vi "Window Comparison.vi"() -> ()   [LabVIEW 2010]
doc: "This VI is used to demonstrate the effect of different window functions upon the spectral leakage and low power freqency components of a signal."
uses:
  <vilib>/Analysis/4window.llb/windowTd.ctl
  <vilib>/measure/maspectr.llb/FFT Power Spectrum for N Chan.vi
  <vilib>/measure/NI_MAPro.lvlib
  <vilib>/Analysis/NI_AALPro.lvlib
panel:
  out "Power Spectrum":cluster{"f0":dbl, "df":dbl, "magnitude":dbl[]}[](graph)=[{"f0"=0.0, "df"=1.0, "magnitude"=[-124.1751058373542, -121.13513758298744, -121.04674254070572, -120.90139130147163, -120.70184950660021, -120.4516362912143, -120.15474721632286, -119.81538139357082, -119.43770325848809, -119.02565646304703, -118.58283491900558, -118.11240678765495, -117.61708195919539, -117.0991117628995, -116.56031017833426, -116.00208758694967, -115.42549025871809, -114.83124082124473, -114.21977665062707, -113.59128440951838, -112.94572985272337, -112.28288260850888, -111.60233599546437, -110.90352211751781, -110.18572255543572, -109.44807497004957, -108.68957588923833, -107.90907987456065, -107.10529517249748, -106.27677584755415, -105.42191027644408, -104.53890574697934, -103.62576875027956, -102.68028036961206, -101.69996594374675, -100.68205789832162, -99.62345027411698, -98.5206430009276, -97.36967332386469, -96.16603091496, -94.90455199278048, -93.5792860707239, -92.1833265180739, -90.7085925655272, -89.14554510684852, -87.48281062482066, -85.70667508309265, -83.80038965903157, -81.74319727265596, -79.50893265081362, -77.06394868660806, -74.36393534729245, -71.34882905910446, -67.93423079359103, -63.99595070698343, -59.33964451276823, -53.63348773495808, -46.22884860135584, -35.49862598039451, -12.538597719535238, -3.3068667017160718, -6.4718206580262425, -28.099138539831067, -41.89347763201883, -50.503546856045254, -56.877338492895234, -61.963331522426735, -66.2069680824894, -69.87995537585789, -69.42951944375393, -62.313348426517905, -68.64789111316674, -80.51401763572983, -82.80836943344987, -84.81279857131192, -86.65729225400504, -88.37465396711826, -89.98359184719408, -91.49777512871867, -92.92807128495059, -94.2834408641184, -95.57142153203343, -96.79843898860452, -97.97002633237325, -99.09098728441205, -100.165521673258, -101.1973240562493, -102.18966249313182, -103.14544227261875, -104.06725801235694, -104.95743664052716, -105.81807313810978, -106.6510604744758, -107.4581148423591, -108.24079705696988, -109.00053080261591, -109.73861826993095, -110.45625362163356, -111.15453463886374, -111.83447283746116, -112.49700228807168, -113.14298733692583, -113.77322938535407, -114.38847286548837, -114.9894105215889, -115.5766880932836, -116.15090847961386, -116.71263545156476, -117.26239697121866, -117.80068816515816, -118.32797399671021, -118.84469167010687, -119.35125280119163, -119.84804537868074, -120.33543554231103, -120.81376919508655, -121.28337347152097, -121.74455807294514, -122.19761648788884, -122.64282710653832, -123.08045424111178, -123.51074906186751, -123.93395045607555, -124.35028581883688, -124.75997177970198, -125.1632148746169, -125.56021216445208, -125.95115180889975, -126.33621359494916, -126.71556942981516, -127.08938379504264, -127.45781417102245, -127.82101142978769, -128.1791202007523, -128.53227921375282, -128.88062161485857, -129.22427526570416, -129.56336301902527, -129.89800298045301, -130.22830874930548, -130.55438964584712, -130.87635093206134, -131.19429399733144, -131.50831656127366, -131.81851284256575, -132.12497372712798, -132.42778692495105, -132.7270371169389, -133.0228060950118, -133.31517289129974, -133.60421390401575, -133.89000301319814, -134.17261169109617, -134.4521091078739, -134.72856222806476, -135.0020359079417, -135.27259298004606, -135.54029434084245, -135.8051990277102, -136.0673642984266, -136.32684569329058, -136.58369712500158, -136.83797091414112, -137.08971787479618, -137.3389873620221, -137.5858273315044, -137.83028439067246, -138.07240385123893, -138.31222977771716, -138.54980503079713, -138.78517131635516, -139.01836922222444, -139.24943826165918, -139.478416911193, -139.7053426466115, -139.93025197873203, -140.15318048594614, -140.37416284818175, -140.59323287623275, -140.81042354077957, -141.02576700189334, -141.2392946361118, -141.4510370617037, -141.6610241613996, -141.86928511277793, -142.07584840369356, -142.28074185791914, -142.483992655868, -142.68562735853408, -142.88567191681955, -143.08415170231268, -143.28109151728637, -143.47651561575393, -143.67044771848697, -143.8629110295719, -144.0539282524225, -144.24352160475738, -144.431712831396, -144.61852321890476, -144.80397361171842, -144.98808441974336, -145.1708756360107, -145.35236684339583, -145.5325772323706, -145.71152560552503, -145.8892303949039, -146.06570966571508, -146.24098113376738, -146.41506216755542, -146.58796980481273, -146.75972075422638, -146.93033141296564, -147.09981786390102, -147.26819590045824, -147.43548101168403, -147.60168841453992, -147.76683304143387, -147.93092956156843, -148.09399237373233, -148.25603563199058, -148.41707323198509, -148.57711883559443, -148.73618585914346, -148.89428749748961, -149.0514367127429, -149.20764625749496, -149.36292866143202, -149.51729625611, -149.6707611575352, -149.82333529904795, -149.9750304115177, -150.125858034163, -150.27582953481837, -150.4249560927558, -150.5732487138425, -150.72071823604801, -150.86737532923135, -151.01323049989048, -151.15829409882457, -151.3025763228256, -151.44608720967113, -151.5888366545089, -151.73083441170797, -151.87209009575957, -152.01261317634646, -152.15241299481323, -152.29149875949037, -152.42987955427094, -152.56756433208255, -152.70456192925553, -152.84088106013726, -152.97653032731174, -153.11151820843295, -153.2458530897144, -153.37954322543285, -153.51259678729724, -153.645021827412, -153.77682629940782, -153.90801807014378, -154.03860489156355, -154.16859442078814, -154.297994277555, -154.42681190437577, -154.55505471423885, -154.68273002263447, -154.80984505159046, -154.93640696126272, -155.06242280680107, -155.1878995912301, -155.31284421983273, -155.43726354300745, -155.5611643189456, -155.68455325535066, -155.80743697809953, -155.92982204851444, -156.05171496612618, -156.17312216066736, -156.2940500070311, -156.4145048149012, -156.5344928315363, -156.65402025195718, -156.7730932174993, -156.89171780289058, -157.00990004204607, -157.12764591254404, -157.24496133777103, -157.36185219883018, -157.47832432363407, -157.59438349337324, -157.71003544570368, -157.82528587844814, -157.94014043807178, -158.05460473752296, -158.16868434411612, -158.2823847835679, -158.39571155703294, -158.50867010817984, -158.621265871078, -158.7335042170598, -158.84539050873965, -158.9569300533994, -159.06812815720016, -159.17899006349944, -159.28952100577783, -159.39972618773655, -159.50961078616334, -159.61917994074602, -159.72843878791122, -159.8373924134828, -159.94604591619043, -160.05440432451513, -160.1624726837545, -160.27025601040685, -160.37775930121828, -160.48498753744693, -160.5919456715788, -160.69863865011925, -160.80507140935055, -160.91124884929033, -161.0171758896533, -161.12285740177512, -161.22829828651413, -161.33350338274414, -161.43847757092217, -161.5432256889789, -161.6477525772953, -161.75206307548777, -161.85616199720897, -161.96005417870816, -162.06374442975874, -162.16723755636502, -162.270538396736, -162.37365172534734, -162.47658236739863, -162.57933512730958, -162.6819148077118, -162.78432621977902, -162.88657416961715, -162.9886634783187, -163.09059900120357, -163.19238539686467, -163.2940277286696, -163.395530647562, -163.49689907261245, -163.59813782096313, -163.69925176615436, -163.80024574808377, -163.901124661947, -164.00189337926753, -164.10255679265657, -164.20311979575402, -164.3035873219207, -164.40396429955373, -164.50425568046768, -164.60446638650893, -164.70460143352153, -164.80466578456029, -164.90466445297545, -165.0046024543232, -165.10448481853496, -165.20431665651734, -165.30410293685438, -165.4038488348927, -165.5035594377934, -165.60323986632395, -165.70289527979156, -165.8025308490354, -165.902151751014, -166.00176321081292, -166.10137045679858, -166.20097871960036, -166.30059330525074, -166.4002194740553, -166.4998625659141, -166.59952790049562, -166.69922084209676, -166.79894674812257, -166.8987110446178, -166.99851913465955, -167.09837642826753, -167.1982884040054, -167.29826053310828, -167.3982982866537, -167.49840718821974, -167.59859272778644, -167.69886047166955, -167.79921594423993, -167.89966469275805, -168.00021229453077, -168.10086434194093, -168.20162636701187, -168.30250394388145, -168.4035027068691, -168.5046281860337, -168.60588597566147, -168.70728161197218, -168.80882068148227, -168.91050867688188, -169.0123511118843, -169.1143535166961, -169.21652128779388, -169.31885988465908, -169.42137466391597, -169.52407093732975, -169.6269540104788, -169.7300290787213, -169.8333012583385, -169.936775605551, -170.04045714285007, -170.14435066809898, -170.24846097914164, -170.35279265258796, -170.4573502952991, -170.5621381219311, -170.66716044353166, -170.77242117456504, -170.8779241627027, -170.98367302507282, -171.0896710874559, -171.19592147231293, -171.30242698937437, -171.40919024382862, -171.51621339879216, -171.62349822909803, -171.7310463832929, -171.83885868730476, -171.94693595044146, -172.0552782093128, -172.1638850589407, -172.27275556913153, -172.38188815021238, -172.4912806012415, -172.6009299794752, -172.7108326963813, -172.8209841038539, -172.93137898052328, -173.04201112773544, -173.15287288382228, -173.26395642711663, -173.37525174021863, -173.48674741812613, -173.59843449204186, -173.71029531974932, -173.82231761578305, -173.93448394918724, -174.0467762268345, -174.15917448253055, -174.2716563870087, -174.3841980792969, -174.49677339554017, -174.60935352674574, -174.72190764756215, -174.83440208790205, -174.94680049842688, -175.05906361949218, -175.17114923291192, -175.28301177041908, -175.39460235009932, -175.50586861988745, -175.61675437167378, -175.72720036139748, -175.83714085932564, -175.9465098365045, -176.05523352274193, -176.16323542842218, -176.27043392042825, -176.37674283974602, -176.48207122634807, -176.58632306032052, -176.68939757067312, -176.7911891428206, -176.89158682473743, -176.99047519343867, -177.08773376572427, -177.18323739909857, -177.27685664633643, -177.36845759329344, -177.45790256058612, -177.54505022577348, -177.6297560787345, -177.7118731136685, -177.79125208522146, -177.86774250587328, -177.9411930462797, -178.0114525474532, -178.07837080326283, -178.14179937404066, -178.20159270346434, -178.25760899112282, -178.30971131079053, -178.3577686663119, -178.40165697327578, -178.44126020379673, -178.47647129169434, -178.5071931923377, -178.53333978317437, -178.55483669830585, -178.57162196956637, -178.5836467422925, -178.59087583084377]}]
  in  "Frequency 2":dbl(knob)=60.2297 scale=0.0..200.0
  in  "Frequency 1":dbl(knob)=70.0581 scale=0.0..200.0
  in  "Amplitude 2":dbl=1.0
  in  "Amplitude 1":dbl=0.001
  in  "stop":bool
  out "Sine1 + Sine2":dynamicdata(graph)=[{"t0"=timestamp(209885 s since 1904-01-01), "dt"=0.001, "Y"=array[1000 elements], "attributes"=variant("NI_ChannelName"=variant(string "Sine1"), "NI_ExpIsRelativeTime"=variant(bool TRUE), "NI_ExpStartTimeStamp"=variant(timestamp timestamp(3289146816.882773 s since 1904-01-01)), "NI_ExpTimeStamp"=variant(timestamp timestamp(3289356701.882773 s since 1904-01-01)), "NI_ExpXDimension"=variant(string "t"))}]
  in  "window":T1=1 items=["Rectangle"=0, "Hanning"=1, "Hamming"=2, "Blackman Harris"=3, "Blackman exacte"=4, "Blackman"=5, "Profil plat"=6, "B-Harris 4 termes "=7, "B-Harris 7 termes"=8, "Lobe latéral bas"=9, "Blackman Nuttall"=11, "Triangle"=30, "Bartlett-Hanning"=31, "Bohman"=32, "Parzen"=33, "Welch"=34, "Kaiser"=60, "Dolph-Tchebychev"=61, "Gaussienne"=62]
  # "Sine Wave 1"
  # "Sine Wave 2"
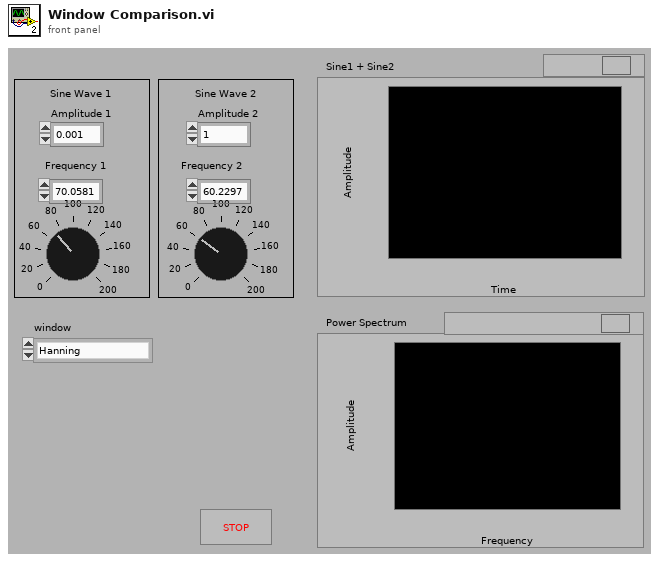
[diagram p1: front panel]
types:
  T1 = typedef "NI_AALPro.lvlib/windowTd.ctl" = u32
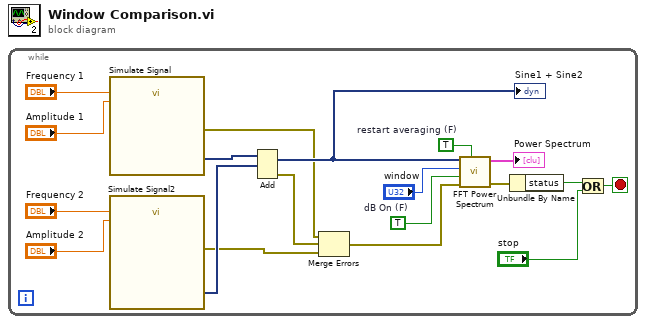
[diagram p0: block diagram]
diagram:
  n1 = while {
    stop <- w6 stop-if-true
    w17 = TRUE  # restart averaging (F)
    w18 = TRUE  # dB On (F)
    n2 = call "Simulate Signal"("Frequency"="Frequency 1", "Amplitude"="Amplitude 1") -> ("Sine1"=w16:dynamicdata, "error out"=w13:errorcluster)  [unwired: 12 in]
    n3 = call "Simulate Signal2"("Frequency"="Frequency 2", "Amplitude"="Amplitude 2") -> ("Sine2"=w15:dynamicdata, "error out"=w11:errorcluster)  [unwired: 12 in]
    n4 = Add(1:w15, 2:w16) -> (0:w14:dynamicdata, 3:w12:errorcluster)  [unwired: 1 in]
    "Sine1 + Sine2" <- w14
    n5 = Merge Errors(w13, w12, w11) -> (w10:errorcluster)
    n6 = call-poly <vilib>:"FFT Power Spectrum.vi"("restart averaging (F)"=w17, "error in (no error)"=w10, "dB On (F)"=w18, "window"="window", "time signals"=w14) -> ("error out"=w9:errorcluster, "power spectra"=→"Power Spectrum":cluster{"f0":dbl, "df":dbl, "magnitude":dbl[]}[])  [unwired: 3 in, 2 out]
    n7 = Unbundle By Name(w9) -> ("status"=w8:bool)
    n8 = Or(x=w8, y="stop") -> (x .or. y?=w6:bool)
  }
